vi "Initialize Daemon.vi"(8 "error in":errorcluster, 9 "Data Model":refnum<class "Device Data Model.lvclass">, 10 "transmission data unit":refnum<class "Transmission Data Unit.lvclass">, 11 "network slave in":refnum<class "Network Slave.lvclass">) -> (0 "error out":errorcluster, 3 "network slave out":refnum<class "Network Slave.lvclass">)   [LabVIEW 2021, in "Network Slave.lvclass"]
doc: "This provides an interface for the slave to launch a protocol daemon."
uses:
  Network Slave.lvclass
  Data Model/Device Data Model.lvclass
  daemon status cluster.ctl
  daemon status.ctl
  Network Slave.lvclass/Network Slave.ctl
  Transmission Data Unit/Transmission Data Unit.lvclass
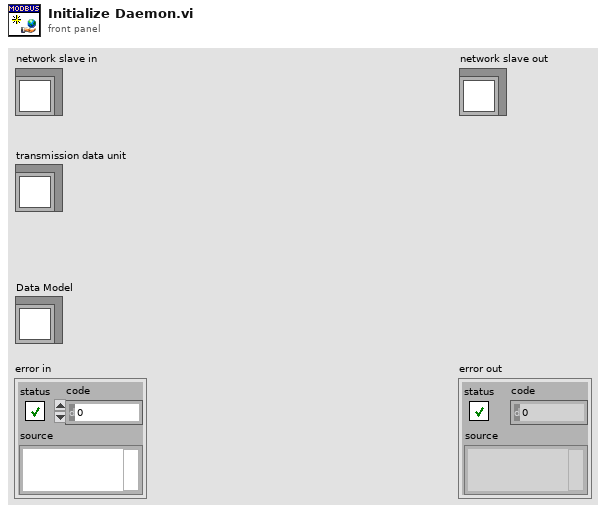
[diagram p1: front panel]
types:
  T1 = typedef "Network Slave.lvclass/daemon status cluster.ctl" = cluster{"error":errorcluster, "status":T2}
  T2 = typedef "Network Slave.lvclass/daemon status.ctl" = enum16{"Not Started", "Running", "Error", "Stopped"}
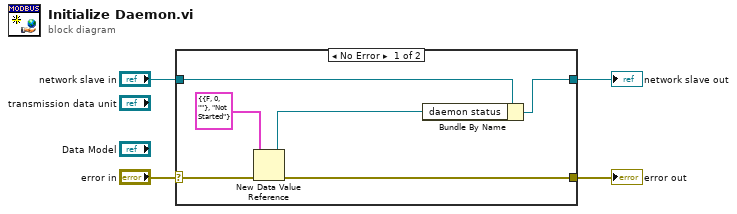
[diagram p0: block diagram]
diagram:
  n1 = case shown="No Error" "error in" {
    selector: "error in" -> [w7 w12]
    tunnel: "network slave in" -> [w10 w11]
    tunnel: [w9 w11] -> w2
    tunnel: [w5 w12] -> w1
    frame No Error {
      n2 = New Data Value Reference(data value=T1 {"error"={"status"=FALSE, "code"=0, "source"=""}, "status"=enum."Not Started"} ("Status"), error in=w7) -> (data value reference=w8:refnum<data-value>, error out=w5:errorcluster)
      n3 = Bundle By Name(cluster=w10, "daemon status"=w8) -> (w9:refnum<class "Network Slave.lvclass">)
    }
    frame Error {
    }
  }
  "error out" <- w1
  "network slave out" <- w2
